vi "_Demagnetization.vi"(8 "demag":T1={"Start(mA)"=40.0, "Time(ms)"=100.0, "step"=1.0}, 11 "Bias_LO_equip":T2={"Node address"=19, "CAN Interface"="CAN0", "Cartridge band"=10, "Slave Node in"={"Address"=19, "Serial Number"=[16, 71, 55, 76, 1, 8, 0, -15]}, "ObjHandle out"=89653312, "POL"=1, "sb"=1, "GPIB_SM (SIS S,V)"="24", "GPIB_DMM (SIS I)"="22", "GPIB_SM (MAG I) "="25", "GPIB_SG(LO)"="19", "GPIB_PW (PAMP) "="6", "GPIB_TMP1(8ch)"="12", "GPIB_TMP2(2ch)  "="13", "WCA_avg"=10, "Rsen"=10.0, "BiasModule"=1, "LOModule "=1, "WCA_LO_FREQ_SET"={"YTO Low freq. [GHz]"=14.42, "YTO High freq. [GHz]"=17.7, "Kvco"=1, "Lock Pol."=0, "SET LO FREQ"=72.5, "Multiplier"=6.0, "YTO (HEX)"=0, "YTO coarse( FREQ)"=25.0, "NULL PLL INTEGRATOR"=FALSE}, "Res for"=0} {"Res for" items=["none", "series res", "parallel res"]; "WCA_LO_FREQ_SET"."YTO coarse( FREQ)" min=25 max=150 step=0.0001 format="%.3f"; "WCA_LO_FREQ_SET"."Multiplier" min=3 max=6 step=3; "WCA_LO_FREQ_SET"."SET LO FREQ" min=25 max=150 step=0.0001 format="%.3f"; "WCA_LO_FREQ_SET"."Lock Pol." items=["Lower", "Upper"]; "WCA_LO_FREQ_SET"."Kvco" items=["7.5MHz/V", "15MHz/V"]; "WCA_LO_FREQ_SET"."YTO High freq. [GHz]" format="%.3f"; "WCA_LO_FREQ_SET"."YTO Low freq. [GHz]" format="%.3f"; "LOModule" items=["Manual", "B10Lab LO", "WCA LO"]; "BiasModule" items=["B10Lab Bias", "WCA BiasModule"]; "Slave Node in"."Serial Number" format="%.0x"; "Slave Node in"."Address" format="%.0x"; "Cartridge band" max=10 step=1; "Node address" format="%.0x"}) -> ()   [LabVIEW 2017]
uses:
  __sub_vi/WCA_NAOJ_sub_vi/WCA_Global.vi
panel:
  out "Link済み":bool=TRUE
  out "current":dbl
  # "LO freq. [GHz]"
  # "YTO LOW\n/High Freq."
  # "ZERO Intgrtr"
  # "Node Address"
  # "Serial Number"
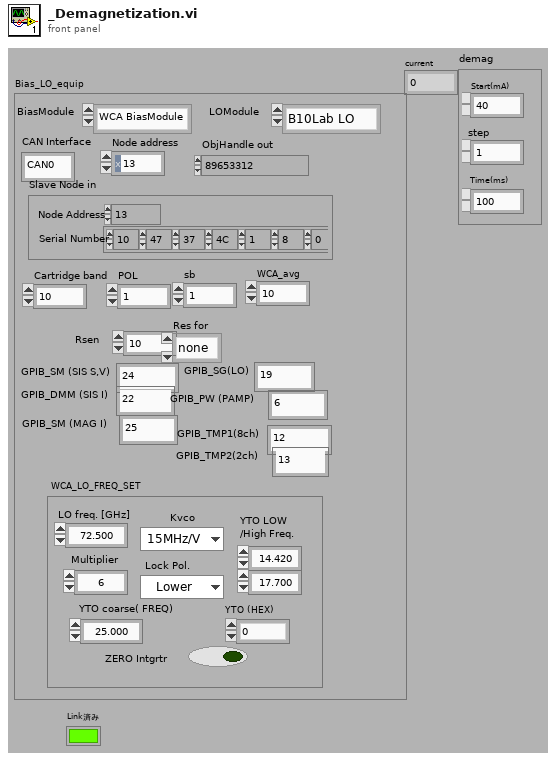
[diagram p1: front panel]
types:
  T1 = cluster{"Start(mA)":dbl, "Time(ms)":dbl, "step":dbl}
  T2 = cluster{"Node address":u16, "CAN Interface":string, "Cartridge band":u32, "Slave Node in":cluster{"Address":i16, "Serial Number":i8[]}, "ObjHandle out":u32, "POL":u32, "sb":u32, "GPIB_SM (SIS S,V)":string, "GPIB_DMM (SIS I)":string, "GPIB_SM (MAG I) ":string, "GPIB_SG(LO)":string, "GPIB_PW (PAMP) ":string, "GPIB_TMP1(8ch)":string, "GPIB_TMP2(2ch)  ":string, "WCA_avg":i32, "Rsen":dbl, "BiasModule":u16, "LOModule ":u16, "WCA_LO_FREQ_SET":cluster{"YTO Low freq. [GHz]":sgl, "YTO High freq. [GHz]":sgl, "Kvco":u16, "Lock Pol.":u16, "SET LO FREQ":sgl, "Multiplier":sgl, "YTO (HEX)":u16, "YTO coarse( FREQ)":sgl, "NULL PLL INTEGRATOR":bool}, "Res for":u16}
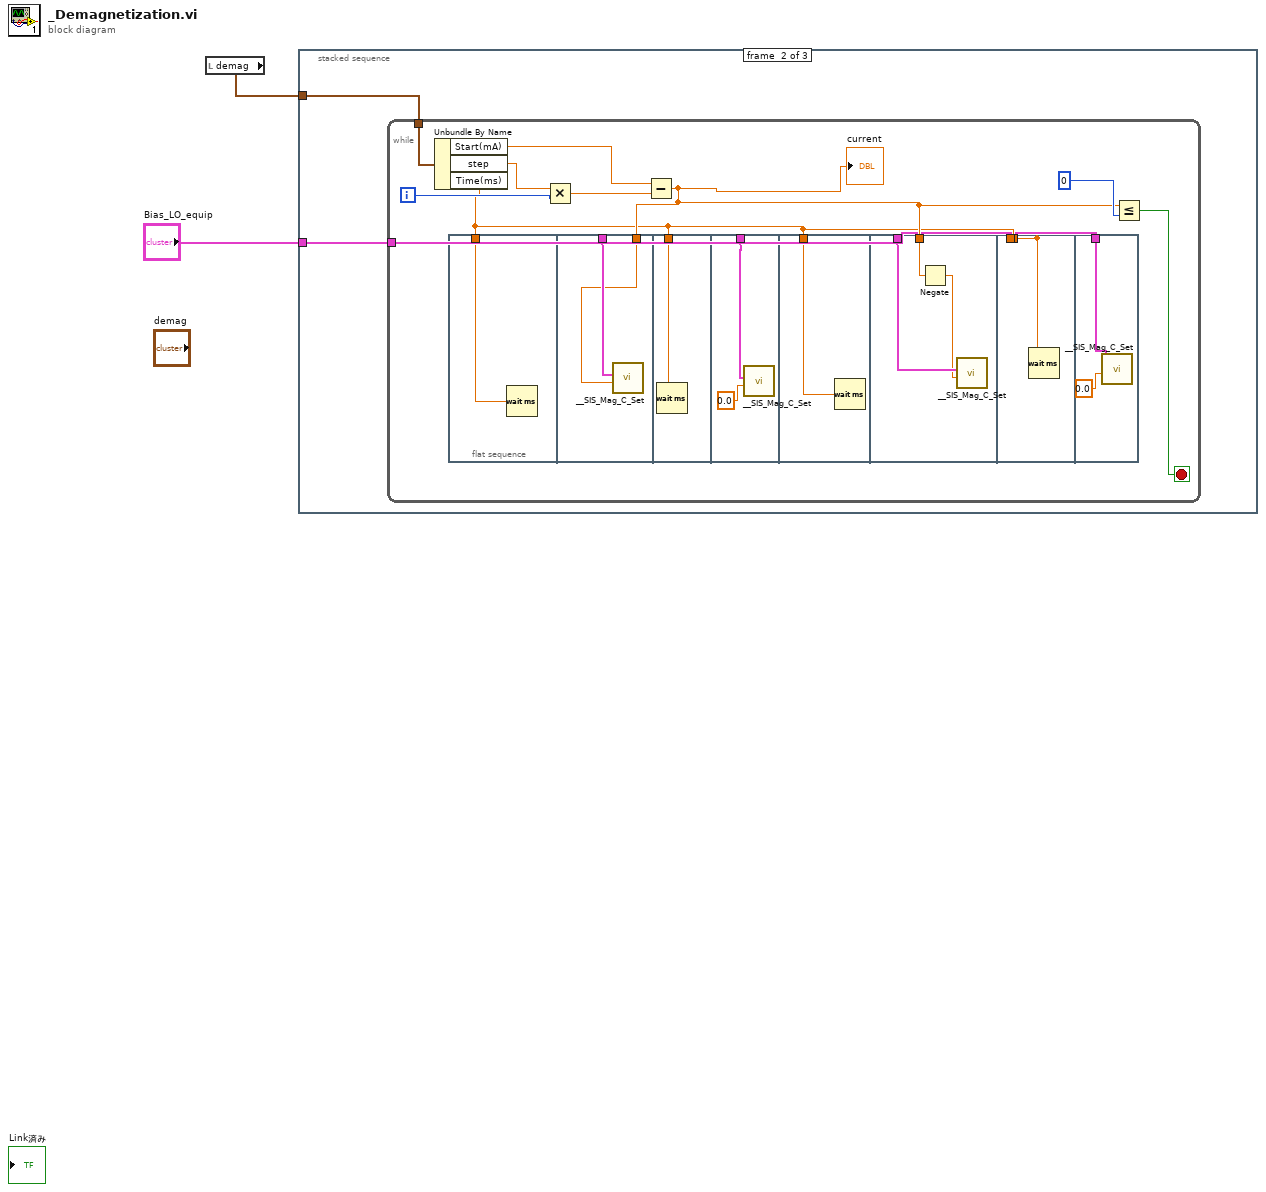
[diagram p0: block diagram]
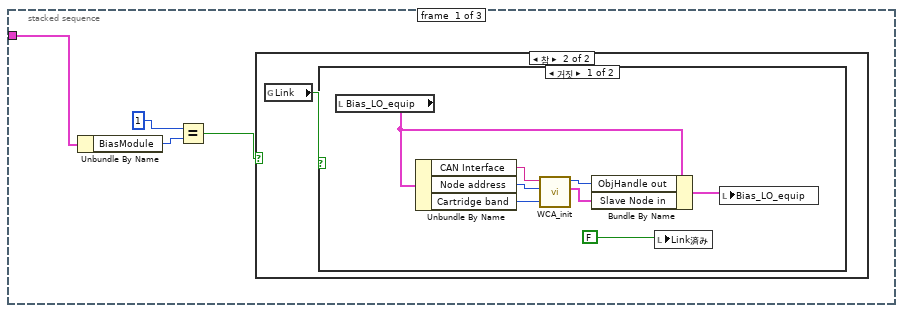
[diagram p2: hidden frame]
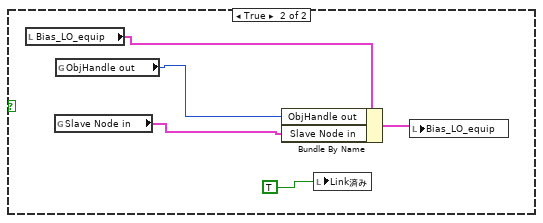
[diagram p4: hidden frame]
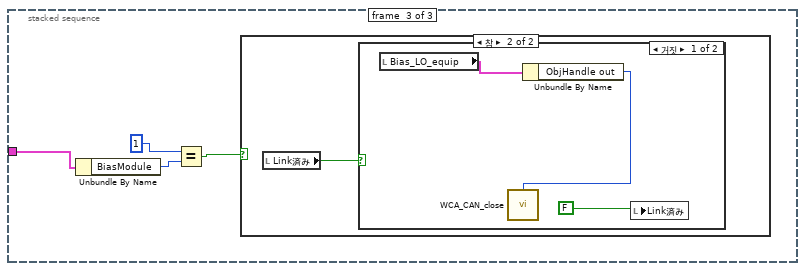
[diagram p5: hidden frame]
diagram:
  n1 = local read "demag"() -> (w2:T1)
  n2 = stacked-sequence {
    tunnel: w2 -> [_ w22 _]
    tunnel: "Bias_LO_equip" -> [w4 w21 w46]
    frame #0 {
      n3 = Unbundle By Name(w4) -> ("BiasModule"=w5:u16)
      n4 = Equal?(x=1, y=w5) -> (x = y?=w3:bool)
      n5 = case shown="참" w3 {
        frame False {
        }
        frame True {
          n6 = global read "WCA_Global.vi" "Link"() -> (w7:bool)
          n7 = case shown="거짓" w7 {
            frame False {
              n8 = local read "Bias_LO_equip"() -> (w8:T2)
              n9 = Unbundle By Name(w8) -> ("CAN Interface"=w12:string, "Node address"=w11:u16, "Cartridge band"=w10:u32)
              n10 = call "WCA_init.vi"("Cartridge band"=w10, "Node address"=w11, "CAN Interface"=w12) -> ("Slave Node in"=w14:cluster{"Address":i16, "Serial Number":i8[]}, "ObjHandle out"=w15:u32)  [unwired: 4 in, 3 out]
              n11 = Bundle By Name(cluster=w8, "ObjHandle out"=w15, "Slave Node in"=w14) -> (w9:T2)
              n12 = local write "Link済み"(FALSE) -> ()
              n13 = local write "Bias_LO_equip"(w9) -> ()
            }
            frame True {
              n14 = local read "Bias_LO_equip"() -> (w19:T2)
              n15 = global read "WCA_Global.vi" "Slave Node in"() -> (w17:cluster{"Address":i16, "Serial Number":i8[]})
              n16 = global read "WCA_Global.vi" "ObjHandle out"() -> (w18:u32)
              n17 = Bundle By Name(cluster=w19, "ObjHandle out"=w18, "Slave Node in"=w17) -> (w20:T2)
              n18 = local write "Link済み"(TRUE) -> ()
              n19 = local write "Bias_LO_equip"(w20) -> ()
            }
          }
        }
      }
    }
    frame #1 {
      n20 = while {
        tunnel: w22 -> [w31]
        tunnel: w21 -> [w23]
        i -> [w29]
        stop <- w25 stop-if-true
        n21 = Unbundle By Name(w31) -> ("Start(mA)"=w28:dbl, "step"=w30:dbl, "Time(ms)"=w24:dbl)
        n22 = flat-sequence {
          tunnel: w24 -> [w33]
          tunnel: w26 -> [w34]
          tunnel: w23 -> [w35]
          tunnel: w24 -> [w36]
          tunnel: w23 -> [w38]
          tunnel: w24 -> [w39]
          tunnel: w26 -> [w42]
          tunnel: w23 -> [w41]
          tunnel: w24 -> [w43]
          tunnel: [w43] -> _
          tunnel: w23 -> [w44]
          frame #0 {
            n23 = Wait (ms)(milliseconds to wait=w33) -> ()  [unwired: 1 out]
          }
          frame #1 {
            n24 = call "__SIS_Mag_C_Set.vi"("Set_Mag_C"=w34, "Bias_LO_equip"=w35) -> ()  [unwired: 10 in]
          }
          frame #2 {
            n25 = Wait (ms)(milliseconds to wait=w36) -> ()  [unwired: 1 out]
          }
          frame #3 {
            n26 = call "__SIS_Mag_C_Set.vi"("Set_Mag_C"=0.0, "Bias_LO_equip"=w38) -> ()  [unwired: 10 in]
          }
          frame #4 {
            n27 = Wait (ms)(milliseconds to wait=w39) -> ()  [unwired: 1 out]
          }
          frame #5 {
            n28 = Negate(x=w42) -> (-x=w40:dbl)
            n29 = call "__SIS_Mag_C_Set.vi"("Set_Mag_C"=w40, "Bias_LO_equip"=w41) -> ()  [unwired: 10 in]
          }
          frame #6 {
            n30 = Wait (ms)(milliseconds to wait=w43) -> ()  [unwired: 1 out]
          }
          frame #7 {
            n31 = call "__SIS_Mag_C_Set.vi"("Set_Mag_C"=0.0, "Bias_LO_equip"=w44) -> ()  [unwired: 10 in]
          }
        }
        n32 = Multiply(x=w30, y=w29) -> (x*y=w32:dbl)
        n33 = Subtract(x=w28, y=w32) -> (x-y=w26:dbl)
        "current" <- w26
        n34 = Less Or Equal?(x=w26, y=0) -> (x <= y?=w25:bool)
      }
    }
    frame #2 {
      n35 = Unbundle By Name(w46) -> ("BiasModule"=w47:u16)
      n36 = Equal?(x=1, y=w47) -> (x = y?=w49:bool)
      n37 = case shown="참" w49 {
        frame False {
        }
        frame True {
          n38 = local read "Link済み"() -> (w50:bool)
          n39 = case shown="거짓" w50 {
            frame False {
              n40 = local read "Bias_LO_equip"() -> (w52:T2)
              n41 = Unbundle By Name(w52) -> ("ObjHandle out"=w51:u32)
              n42 = call "WCA_CAN_close.vi"("ObjHandle in"=w51) -> ()  [unwired: 14 in, 1 out]
              n43 = local write "Link済み"(FALSE) -> ()
            }
            frame True {
            }
          }
        }
      }
    }
  }
